vi "test_TrajectoryDL090201FrameScan.vi"() -> ()   [LabVIEW 2010, in "TrajectoryDL090201FrameScan.lvclass"]
uses:
  TrajectoryDL090201FrameScan.lvclass
  TrajectoryDL091126GenericVoxel/TrajectoryDL091126GenericVoxel/transformation_parameters.ctl
  common/classes/SpaceVector/SpaceVector/SpaceVector.lvclass
  common/classes/ErrorController/ErrorController/ErrorController.lvclass
  common/enumerations/functional_global_action_enum.ctl
  common/classes/ErrorController/ErrorController/class_data.vi
  common/classes/Box/Box/Box.lvclass
  TrajectoryDL091126GenericVoxel/TrajectoryDL091126GenericVoxel/TrajectoryDL091126GenericVoxel.lvclass
panel:
  out "error handler loaded?":bool
  in  "stop":bool
  in  "create button":bool
  in  "rotate":dbl[unit](slide)
  in  "zoom":dbl(slide)=1.0 min=1.0 scale=1.0..10.0
  in  "tilt":dbl[unit](slide)
  out "time for transformation [ms]":u32
  in  "scattering length":dbl[unit]=0.00019999999999999998
  in  "modifier base value":dbl=1.0
  in  "initialise":bool
  in  "x resolution":i32=256
  in  "y resolution":i32=256
  in  "x ratio factor":dbl=1.0
  in  "y ratio factor":dbl=1.0
  in  "x dimension":dbl[unit]=9.999999999999999e-05
  in  "y dimension":dbl[unit]=9.999999999999999e-05
  in  "z dimension":dbl[unit]=9.999999999999999e-05
  out "scanner values":dbl[][](graph)
  out "modifier values":dbl[](graph)
  # "Test TrajectoryDL090201FrameScan"
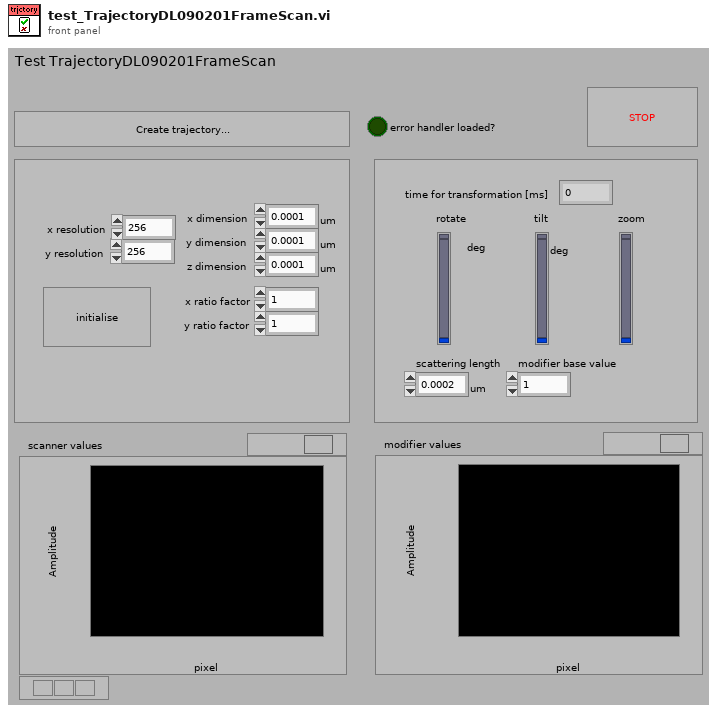
[diagram p1: front panel]
types:
  T1 = typedef "TrajectoryDL091126GenericVoxel.lvclass/transformation_parameters.ctl" = cluster{"scale factor":dbl, "rotation angle":dbl[unit], "tilting angle":dbl[unit], "offset":refnum<class "SpaceVector.lvclass">}
  T2 = typedef "functional_global_action_enum.ctl" = enum16{"get", "set", "reset"}
  T3 = typedef "plugin_specification.ctl" = cluster{"class path":string, "configuration":string, "label":string, "settings name":string}
  T4 = typedef "XComponentSpecification.xctl/data.ctl" = cluster{"class path":string, "configuration":string, "label":string, "settings name":string}
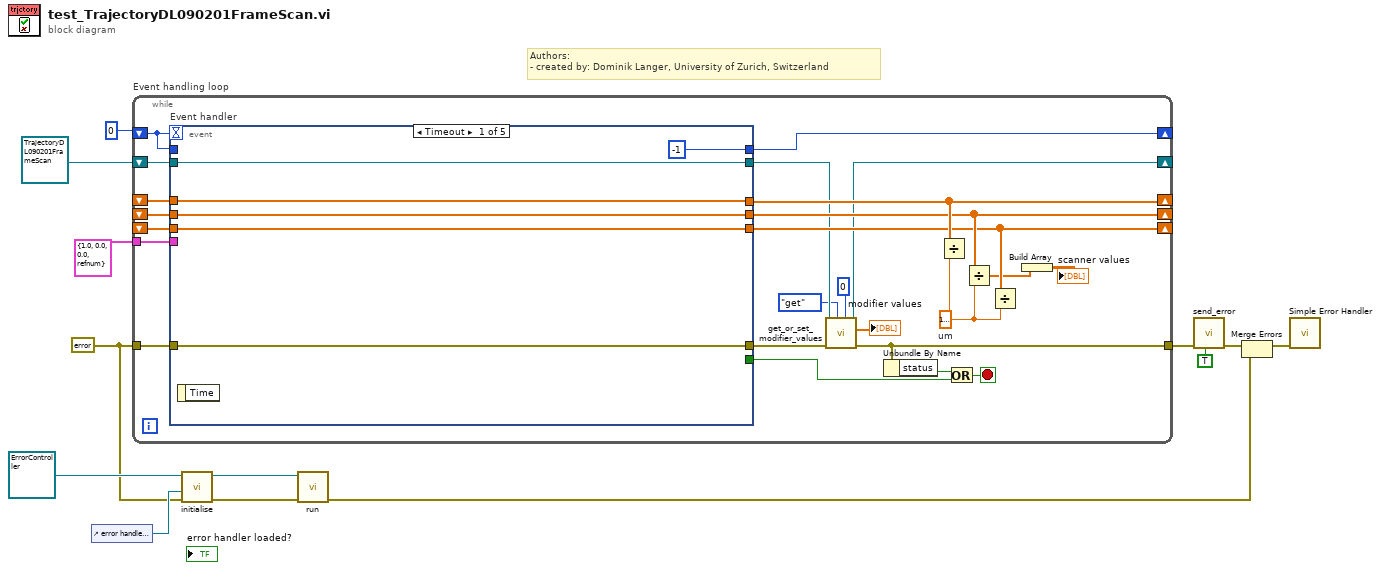
[diagram p0: block diagram]
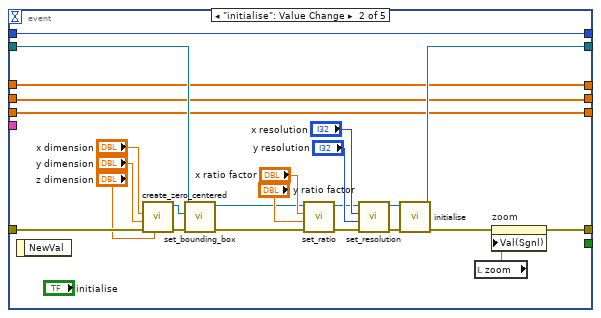
[diagram p2: hidden frame]
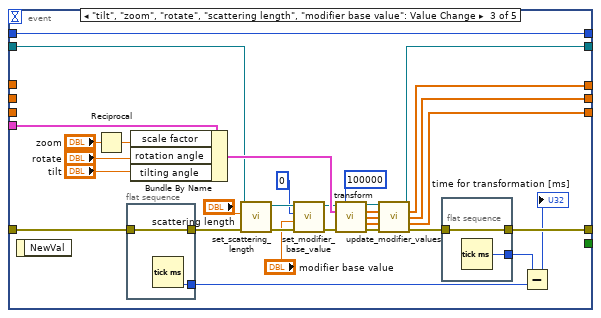
[diagram p3: hidden frame]
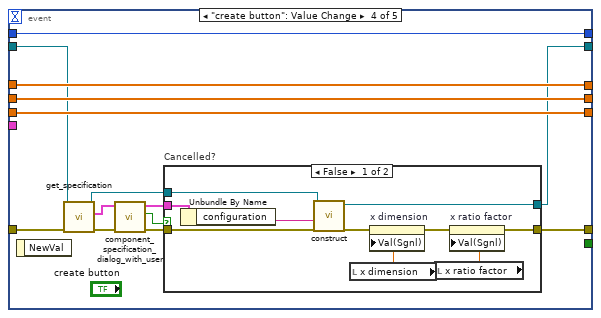
[diagram p4: hidden frame]
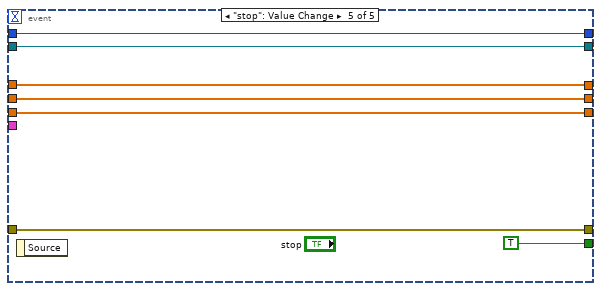
[diagram p6: hidden frame]
diagram:
  w6 = errorcluster {"status"=FALSE, "code"=0, "source"=""} ("error out")
  # "Authors: \n- created by: Dominik Langer, University of Zurich, Switzerland"
  n1 = control-ref of="error handler loaded?"() -> (w7:refnum<vi>)
  n2 = while "Event handling loop" {
    shift-right: [w19] -> _
    shift-left: 0 -> [w36]
    shift-right: [w24] -> _
    shift-left: refnum<class "TrajectoryDL090201FrameScan.lvclass"> refnum ("TrajectoryDL090201FrameScan.lvclass") -> [w35]
    tunnel: T1 {"scale factor"=1.0, "rotation angle"=0.0, "tilting angle"=0.0, "offset"=refnum} ("transformation parameters") -> [w34]
    shift-right: [w30] -> _
    shift-left: _ -> [w33]
    shift-right: [w27] -> _
    shift-left: _ -> [w32]
    shift-right: [w26] -> _
    shift-left: _ -> [w31]
    tunnel: w6 -> [w37]
    tunnel: [w18] -> w5
    stop <- w16 stop-if-true
    w29 = dbl[unit] 1e-06  # um
    n3 = event "Event handler" shown="[0] Timeout" {
      selector: _ -> [_ _ _ _ _]
      dyn-events: _ -> [_ _ _ _ _]
      timeout: w36 -> [_ _ _ _ _]
      tunnel: w37 -> [w38 w67 w93 w111 w137]
      tunnel: [w38 w45 w92 w114 w137] -> w25
      tunnel: w36 -> [_ w68 w100 w118 w136]
      tunnel: [-1 w68 w100 w118 w136] -> w19
      tunnel: [w39 w63 w83 w106 w135] -> w23
      tunnel: w35 -> [w39 w64 w76 w108 w135]
      tunnel: [_ _ _ _ TRUE] -> w15
      tunnel: w34 -> [_ _ w99 _ _]
      tunnel: w33 -> [w42 w58 _ w117 w133]
      tunnel: [w42 w58 w80 w117 w133] -> w30
      tunnel: [w41 w57 w79 w116 w132] -> w27
      tunnel: [w40 w56 w78 w115 w131] -> w26
      tunnel: w32 -> [w41 w57 _ w116 w132]
      tunnel: w31 -> [w40 w56 _ w115 w131]
      event Timeout {
        n4 = event-data() -> ()  [unwired: 2 out]
      }
      event "initialise": Value Change {
        n5 = event-data() -> ()  [unwired: 2 out]
        n6 = call "create_zero_centered.vi"("z dimension"="z dimension", "error in (no error)"=w67, "y dimension"="y dimension", "x dimension"="x dimension") -> ("error out"=w66:errorcluster, "Box out"=w65:refnum<class "Box.lvclass">)  [unwired: 6 out]
        n7 = call-dynamic "set_bounding_box.vi"("error in (no error)"=w66, "Box.lvclass"=w65, "GenericTrajectory in"=w64) -> ("error out"=w52:errorcluster, "GenericTrajectory out"=w51:refnum<class "TrajectoryDL090201FrameScan.lvclass">)  [unwired: 7 out]
        n8 = call-dynamic "set_ratio.vi"("error in (no error)"=w52, "y"="y ratio factor", "x"="x ratio factor", "TrajectoryDL090201FrameScan in"=w51) -> ("error out"=w53:errorcluster, "TrajectoryDL090201FrameScan out"=w50:refnum<class "TrajectoryDL090201FrameScan.lvclass">)  [unwired: 6 in]
        n9 = call-dynamic "set_resolution.vi"("error in (no error)"=w53, "y"="y resolution", "x"="x resolution", "TrajectoryDL090201FrameScan in"=w50) -> ("error out"=w62:errorcluster, "TrajectoryDL090201FrameScan out"=w61:refnum<class "TrajectoryDL090201FrameScan.lvclass">)  [unwired: 6 out]
        n10 = call-dynamic "initialise.vi"("error in (no error)"=w62, "DL090201FrameScanTrajectory in"=w61) -> ("error out"=w46:errorcluster, "DL090201FrameScanTrajectory out"=w63:refnum<class "TrajectoryDL090201FrameScan.lvclass">)  [unwired: 8 out]
        n11 = local read "zoom"() -> (w44:dbl)
        n12 = property on="zoom" class="Slide (strict)"(error in=w46, "Val(Sgnl)"=w44) -> (error out=w45:errorcluster)  [unwired: 1 in, 1 out]
      }
      event "tilt", "zoom", "rotate", "scattering length", "modifier base value": Value Change {
        n13 = event-data() -> ()  [unwired: 2 out]
        n14 = Reciprocal(x="zoom") -> (1/x=w94:dbl)
        n15 = flat-sequence {
          tunnel: w93 -> [w104]
          tunnel: [w104] -> w77
          tunnel: [w103] -> w90
          frame #0 {
            n16 = Tick Count (ms)() -> (millisecond timer value=w103:u32)
          }
        }
        n17 = Bundle By Name(cluster=w99, "scale factor"=w94, "rotation angle"="rotate", "tilting angle"="tilt") -> (w96:T1)
        n18 = call-dynamic "set_scattering_length.vi"("error in (no error)"=w77, "scattering length"="scattering length", "GenericTrajectory.lvclass in"=w76) -> ("error out"=w74:errorcluster, "GenericTrajectory.lvclass out"=w72:refnum<class "TrajectoryDL090201FrameScan.lvclass">)  [unwired: 7 in]
        n19 = call-dynamic "set_modifier_base_value.vi"("error in (no error)"=w74, "modifier base value"="modifier base value", "modifier index"=0, "GenericTrajectory.lvclass in"=w72) -> ("error out"=w73:errorcluster, "GenericTrajectory.lvclass out"=w69:refnum<class "TrajectoryDL090201FrameScan.lvclass">)  [unwired: 6 in]
        n20 = call-dynamic "transform.vi"("GenericTrajectory in"=w69, "block size"=100000, "transformation parameters"=w96, "error in (no error)"=w73) -> ("GenericTrajectory out"=w84:refnum<class "TrajectoryDL090201FrameScan.lvclass">, "x coordinates"=w85:dbl[unit][], "y coordinates"=w82:dbl[unit][], "z coordinates"=w81:dbl[unit][], "error out"=w87:errorcluster)  [unwired: 7 in]
        n21 = call-dynamic "update_modifier_values.vi"("TrajectoryDL091126GenericVoxel in"=w84, "x coordinates in"=w85, "y coordinates in"=w82, "z coordinates in"=w81, "error in (no error)"=w87) -> ("TrajectoryDL091126GenericVoxel out"=w83:refnum<class "TrajectoryDL090201FrameScan.lvclass">, "x coordinates out"=w80:dbl[unit][], "y coordindates out"=w79:dbl[unit][], "z coordinates out"=w78:dbl[unit][], "error out"=w86:errorcluster)  [unwired: 6 in]
        n22 = flat-sequence {
          tunnel: w86 -> [w102]
          tunnel: [w102] -> w92
          tunnel: [w101] -> w91
          frame #0 {
            n23 = Tick Count (ms)() -> (millisecond timer value=w101:u32)
          }
        }
        n24 = Subtract(x=w91, y=w90) -> (x-y=→"time for transformation [ms]":u32)
      }
      event "create button": Value Change {
        n25 = event-data() -> ()  [unwired: 2 out]
        n26 = call-dynamic "get_specification.vi"("error in (no error)"=w111, "GenericPlugin in"=w108) -> ("error out"=w110:errorcluster, "component specification"=w109:T3, "GenericPlugin out"=w107:refnum<class "TrajectoryDL090201FrameScan.lvclass">)  [unwired: 6 in, 1 out]
        n27 = call "component_specification_dialog_with_user.vi"("error in (no error)"=w110, "component specification in"=w109) -> ("error out"=w113:errorcluster, "cancelled?"=w105:bool, "component specification out"=w112:T4)  [unwired: 7 in]
        n28 = case "Cancelled?" shown="False" w105 {
          tunnel: [w124 w130] -> w114
          tunnel: w113 -> [w123 w130]
          tunnel: w112 -> [w122 _]
          tunnel: w107 -> [w120 w129]
          tunnel: [w119 w129] -> w106
          frame False {
            n29 = Unbundle By Name(w122) -> ("configuration"=w121:string)
            n30 = call-dynamic "construct.vi"("error in (no error)"=w123, "configuration name"=w121, "GenericPlugin in"=w120) -> ("error out"=w125:errorcluster, "GenericPlugin out"=w119:refnum<class "TrajectoryDL090201FrameScan.lvclass">)  [unwired: 7 in]
            n31 = local read "x dimension"() -> (w128:dbl[unit])
            n32 = property on="x dimension" class="DigNum (strict)"(error in=w125, "Val(Sgnl)"=w128) -> (error out=w127:errorcluster)  [unwired: 1 in, 1 out]
            n33 = local read "x ratio factor"() -> (w126:dbl)
            n34 = property on="x ratio factor" class="DigNum (strict)"(error in=w127, "Val(Sgnl)"=w126) -> (error out=w124:errorcluster)  [unwired: 1 in, 1 out]
          }
          frame True {
          }
        }
      }
      event "stop": Value Change {
        n35 = event-data() -> ()  [unwired: 2 out]
      }
    }
    n36 = call-dynamic "get_or_set_modifier_values.vi"("modifier index"=0, "action"=functional_global_action_enum."get", "error in (no error)"=w25, "GenericTrajectory in"=w23) -> ("error out"=w18:errorcluster, "modifier values out"=→"modifier values":dbl[], "GenericTrajectory out"=w24:refnum<class "TrajectoryDL090201FrameScan.lvclass">)  [unwired: 5 in]
    n37 = Unbundle By Name(w18) -> ("status"=w17:bool)
    n38 = Divide(x=w30, y=w29) -> ()  [unwired: 1 out]
    n39 = Or(x=w17, y=w15) -> (x .or. y?=w16:bool)
    n40 = Divide(x=w27, y=w29) -> (x/y=w14:dbl[])
    n41 = Divide(x=w26, y=w29) -> ()  [unwired: 1 out]
    n42 = Build Array(w14) -> (→"scanner values":dbl[][])
  }
  n43 = call-dynamic "initialise.vi"("error in (no error)"=w6, "error boolean"=w7, "ErrorController in"=refnum<class "ErrorController.lvclass"> refnum ("ErrorController.lvclass")) -> ("error out"=w8:errorcluster, "ErrorController out"=w9:refnum<class "ErrorController.lvclass">)  [unwired: 7 in]
  n44 = call "run.vi"("error in (no error)"=w8, "ErrorController in"=w9) -> ("error out"=w1:errorcluster)  [unwired: 8 in, 1 out]
  n45 = call "send_error.vi"("last error? (F)"=TRUE, "error in (no error)"=w5) -> ("error out"=w3:errorcluster)  [unwired: 9 in]
  n46 = Merge Errors(w3, w1) -> (w2:errorcluster)
  n47 = call <vilib>:"Simple Error Handler.vi"("error in (no error)"=w2) -> ()  [unwired: 4 in, 5 out]
